vi "Cache_Members Global.vi"() -> ()   [LabVIEW 2020, in "ClassLoader.lvlib"]
uses:
  ClassLoader.lvlib
  Ctl/Ctl_Member Map.ctl
  <vilib>/Utility/Data Type/Member VI Info.ctl
panel:
  in  "Members":map{string, T1}(c390)
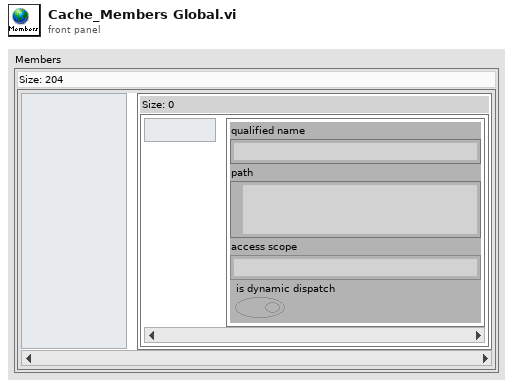
[diagram p1: front panel]
types:
  T1 = typedef "ClassLoader.lvlib/Ctl_Member Map.ctl" = map{string, T2}
  T2 = typedef "Member VI Info.ctl" = cluster{"qualified name":string, "path":path, "access scope":enum32{"invalid scope", "public", "private", "protected", "community"}, "is dynamic dispatch":bool}
diagram:
